vi "rozklad wyslanej ramki jazda.vi"(11 "Wyslany":string) -> (0 "obrotjazda":dbl, 1 "hamowanie":bool, 2 "skretjazda":dbl, 3 "pwmjazda":dbl, 6 "hamowaniejazda":dbl)   [LabVIEW 2015]
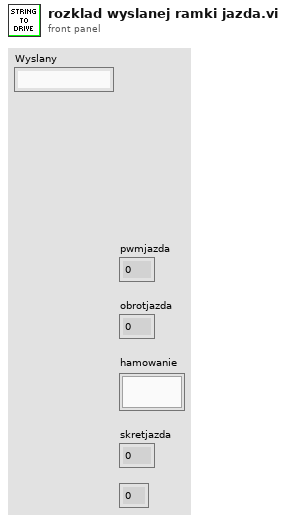
[diagram p1: front panel]
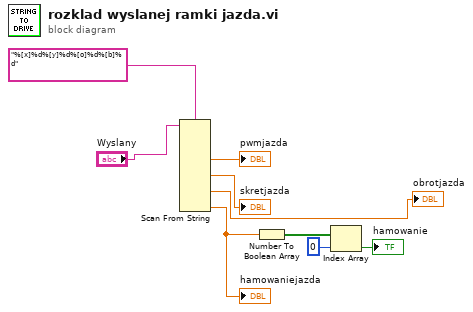
[diagram p0: block diagram]
diagram:
  n1 = Scan From String(format string="%[x]%d%[y]%d%[o]%d%[b]%d", input string="Wyslany") -> (output 2=→"pwmjazda":dbl, output 4=→"skretjazda":dbl, output 6=→"obrotjazda":dbl, output 8=w4:dbl)  [unwired: 14 in, 3 out]
  "hamowaniejazda" <- w4
  n2 = Number To Boolean Array(number=w4) -> (Boolean array=w5:bool[])
  n3 = Index Array(array=w5, index=0 ("y")) -> (element=→"hamowanie":bool)
